vi "ALTS-2015 Close All.vi"(8 "error in":errorcluster) -> (0 "error out":errorcluster)   [LabVIEW 2013]
doc: "Copyright © 2005, Soliton Technologies.\nAll rights reserved."
uses:
  Controls/ALTS-2015 Write DB Write Result Driver Cases.ctl
  Controls/ALTS-2015 Obtain Test Data DB Driver Options.ctl
  SLL DAQ Engine/Software/Source Code/Sub VIs/DAQ Engine/Controls/SLL DE DAQ Global Options.ctl
  SLL DAQ Engine/Software/Source Code/Sub VIs/DAQ Engine/Controls/SLL DE DAQ Global Elements.ctl
  Controls/ALTS-2015 Scanner Driver Options.ctl
  Controls/ALTS-2015 LV2GBL Options.ctl
  Controls/ALTS-2015 DB Driver Options.ctl
  SLL DAQ Engine/Software/Source Code/Sub VIs/DAQ Engine/Controls/SLL DE DO Command LV2Global Options.ctl
  OPC Engine/Globals/ALTS-2015 OPC Engine Globals.vi
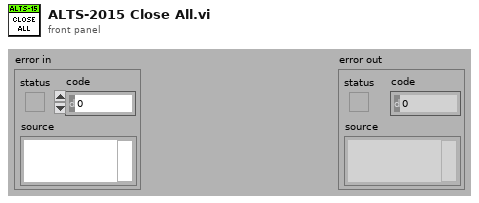
[diagram p1: front panel]
types:
  T1 = typedef "ALTS-2015 DB Driver Options.ctl" = enum16{"Init", "Read DB", "Close"}
  T2 = typedef "ALTS-2015 LV2GBL Options.ctl" = enum16{"Read all", "Write all"}
  T3 = typedef "ALTS-2015 Scanner Driver Options.ctl" = enum16{"Initialize Scanner", "Read Scanner", "Close Scanner"}
  T4 = typedef "SLL DE DAQ Global Elements.ctl" = enum16{"AI Error", "AO Error", "DI Error", "DO Error", "AI Restart", "DI Restart", "AI Running", "AO Running", "DI Running", "DO Running", "DAQ Exit?"}
  T5 = typedef "SLL DE DAQ Global Options.ctl" = enum16{"Init", "Write 1", "Read 1", "Write Array", "Read Array", "Clear"}
  T6 = typedef "ALTS-2015 Obtain Test Data DB Driver Options.ctl" = enum16{"Init", "Read Test Data Results", "Close"}
  T7 = typedef "ALTS-2015 Write DB Write Result Driver Cases.ctl" = enum16{"Init", "Write Result", "Close"}
  T8 = typedef "SLL DE DO Command LV2Global Options.ctl" = enum16{"Init/Register Events", "Get Event Refnum", "Fire Event", "Destroy Event"}
  T9 = typedef "ALTS-2015 INI Configuration Cluster.ctl" = cluster{"Application":cluster{"Rerun Count":i32, "Workorder No":string}, "Station Details":cluster{"Sensor Name 1":string, "Sensor Name 2":string, "Sensor Name 3":string, "Sensor Name 4":string, "Station1 Enable":bool, "Station2 Enable":bool, "Station3 Enable":bool, "Station4 Enable":bool}, "Database":cluster{"Database Connection Link":path, "Result Procedure":string, "User":string, "Password":string, "Prompt":bool, "Station 1 LT Result DB DSN Path":path, "Station 2 LT Result DB DSN Path":path, "Station 3 LT Result DB DSN Path":path, "Station 4 LT Result DB DSN Path":path, "AirLeakTestResult Procedure":string, "Serial Details Procedure":string}, "Simulation":cluster{"Simulate DAQ Hardware":bool, "Simulate Result DB Write":bool, "Simulate Scanner":bool, "Simulate OPC":bool, "Simulate Serial Details DB":bool, "Simulate Result DB":bool, "Simulate Scanner DB Path":path, "Simulate Serial Details DB Path":path, "Simulate Result DB Path":path}, "Barcode Scanner1":cluster{"Scanner IP":string, "Scanner Port":u16, "#Bytes to Read":i32}, "Barcode Scanner2":cluster{"Enabled?":bool, "Scanner IP":string, "Scanner Port":u16, "#Bytes to Read":i32}}
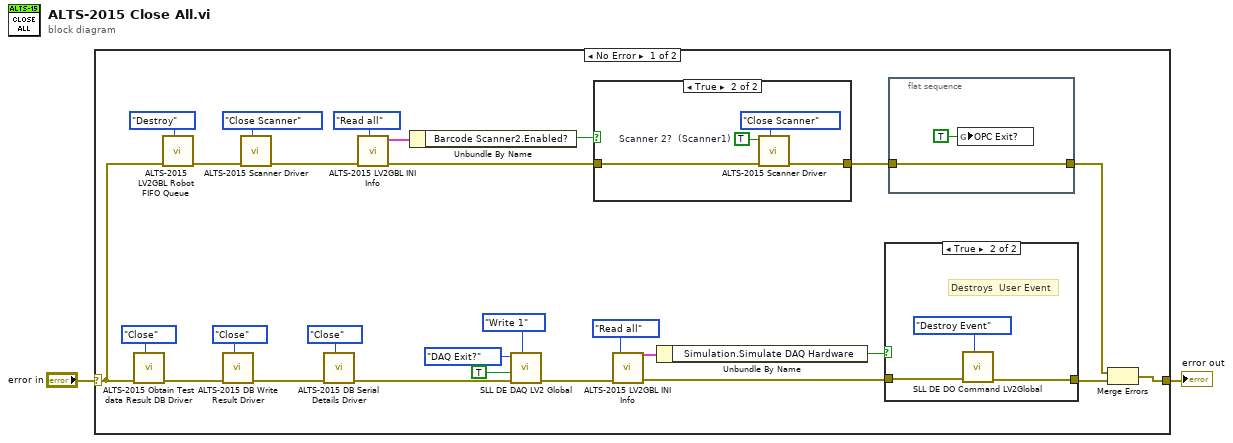
[diagram p0: block diagram]
diagram:
  n1 = case shown="No Error" "error in" {
    selector: "error in" -> [w16 w41]
    tunnel: [w8 w41] -> w1
    frame No Error {
      n2 = call "ALTS-2015 Obtain Test data Result DB Driver.vi"("Option"=ALTS-2015_Obtain_Test_Data_DB_Driver_Options."Close", "error in"=w16) -> ("error out"=w26:errorcluster)  [unwired: 8 in, 1 out]
      n3 = call "ALTS-2015 LV2GBL Robot FIFO Queue.vi"("Enum"=enum16{"Init", "Enqueue", "Dequeue", "Destroy"}."Destroy", "error in (no error)"=w16) -> ("error out"=w9:errorcluster)  [unwired: 7 in, 2 out]
      n4 = call "ALTS-2015 DB Write Result Driver.vi"("Operation"=ALTS-2015_Write_DB_Write_Result_Driver_Cases."Close", "Error In"=w26) -> ("error out"=w6:errorcluster)  [unwired: 9 in]
      n5 = call "ALTS-2015 Scanner Driver.vi"("Operation"=ALTS-2015_Scanner_Driver_Options."Close Scanner", "error in (no error)"=w9) -> ("error out"=w11:errorcluster)  [unwired: 8 in, 1 out]
      n6 = call "ALTS-2015 DB Serial Details Driver.vi"("Operation"=ALTS-2015_DB_Driver_Options."Close", "error in (no error)"=w6) -> ("error out"=w5:errorcluster)  [unwired: 4 in, 5 out]
      n7 = call "ALTS-2015 LV2GBL INI Info.vi"("Options"=ALTS-2015_LV2GBL_Options."Read all", "error in"=w11) -> ("error out"=w13:errorcluster, "Configuration Cluster Out"=w12:T9)  [unwired: 8 in]
      n8 = Unbundle By Name(w12) -> ("Barcode Scanner2.Enabled?"=w14:bool)
      n9 = call "SLL DE DAQ LV2 Global.vi"("Option"=SLL_DE_DAQ_Global_Options."Write 1", "error in (no error)"=w5, "Status In"=TRUE, "Element"=SLL_DE_DAQ_Global_Elements."DAQ Exit?") -> ("error out"=w21:errorcluster)  [unwired: 5 in, 2 out]
      n10 = case shown="True" w14 {
        tunnel: w13 -> [w32 w35]
        tunnel: [w32 w33] -> w4
        frame False {
        }
        frame True {
          w34 = TRUE  # Scanner 2?  (Scanner1)
          n11 = call "ALTS-2015 Scanner Driver.vi"("Operation"=ALTS-2015_Scanner_Driver_Options."Close Scanner", "error in (no error)"=w35, "Scanner 2?  (Scanner1)"=w34) -> ("error out"=w33:errorcluster)  [unwired: 7 in, 1 out]
        }
      }
      n12 = call "ALTS-2015 LV2GBL INI Info.vi"("Options"=ALTS-2015_LV2GBL_Options."Read all", "error in"=w21) -> ("error out"=w23:errorcluster, "Configuration Cluster Out"=w25:T9)  [unwired: 8 in]
      n13 = Unbundle By Name(w25) -> ("Simulation.Simulate DAQ Hardware"=w24:bool)
      n14 = case shown="True" w24 {
        tunnel: w23 -> [w37 w39]
        tunnel: [w37 w40] -> w20
        frame False {
        }
        frame True {
          # "Destroys  User Event"
          n15 = call "SLL DE DO Command LV2Global.vi"("Option"=SLL_DE_DO_Command_LV2Global_Options."Destroy Event", "Error in (no error)"=w39) -> ("Error out"=w40:errorcluster)  [unwired: 8 in, 1 out]
        }
      }
      n16 = flat-sequence {
        tunnel: w4 -> [w30]
        tunnel: [w30] -> w3
        frame #0 {
          n17 = global write "ALTS-2015 OPC Engine Globals.vi" "OPC Exit?"(TRUE ("OPC Exit?")) -> ()
        }
      }
      n18 = Merge Errors(w3, w20) -> (w8:errorcluster)
    }
    frame Error {
    }
  }
  "error out" <- w1
